vi "GetProbePlanCoordinates.vi"(8 "Use index as X coord":bool=TRUE, 9 "Probe Card Channels":i32=1) -> (0 "file path":string, 2 "OK?":bool, 3 "Array":T1(array[cluster]))   [LabVIEW 2018] (continued)
\nLabel=Strip\t763\tX=19403.20\ty=17360.64 \nLabel=Strip\t764\tX=19749.10\ty=17461.35 \nLabel=Strip\t765\tX=19396.46\ty=17516.68 \nLabel=Strip\t766\tX=19742.32\ty=17617.52 \nLabel=Strip\t767\tX=19389.66\ty=17672.72 \nLabel=Strip\t768\tX=19735.48\ty=17773.69 \nLabel=Strip\t769\tX=19382.79\ty=17828.75 \nLabel=Strip\t770\tX=19728.58\ty=17929.86 \nLabel=Strip\t771\tX=19375.87\ty=17984.79 \nLabel=Strip\t772\tX=19721.61\ty=18086.03 \nLabel=Strip\t773\tX=19368.89\ty=18140.82 \nLabel=Strip\t774\tX=19714.59\ty=18242.20 \nLabel=Strip\t775\tX=19361.84\ty=18296.85 \nLabel=Strip\t776\tX=19707.51\ty=18398.36 \nLabel=Strip\t777\tX=19354.74\ty=18452.88 \nLabel=Strip\t778\tX=19700.36\ty=18554.52 \nLabel=Strip\t779\tX=19347.57\ty=18608.91 \nLabel=Strip\t780\tX=19693.16\ty=18710.69 \nLabel=Strip\t781\tX=19340.34\ty=18764.93 \nLabel=Strip\t782\tX=19685.89\ty=18866.85 \nLabel=Strip\t783\tX=19333.06\ty=18920.96 \nLabel=Strip\t784\tX=19678.57\ty=19023.00 \nLabel=Strip\t785\tX=19325.71\ty=19076.98 \nLabel=Strip\t786\tX=19671.18\ty=19179.16 \nLabel=Strip\t787\tX=19318.30\ty=19233.00 \nLabel=Strip\t788\tX=19663.73\ty=19335.32 \nLabel=Strip\t789\tX=19310.84\ty=19389.02 \nLabel=Strip\t790\tX=19656.23\ty=19491.47 \nLabel=Strip\t791\tX=19303.31\ty=19545.04 \nLabel=Strip\t792\tX=19648.66\ty=19647.62 \nLabel=Strip\t793\tX=19295.72\ty=19701.06 \nLabel=Strip\t794\tX=19641.03\ty=19803.77 \nLabel=Strip\t795\tX=19288.07\ty=19857.07 \nLabel=Strip\t796\tX=19633.34\ty=19959.92 \nLabel=Strip\t797\tX=19280.36\ty=20013.08 \nLabel=Strip\t798\tX=19625.59\ty=20116.07 \nLabel=Strip\t799\tX=19272.59\ty=20169.10 \nLabel=Strip\t800\tX=19617.78\ty=20272.22 \nLabel=Strip\t801\tX=19264.76\ty=20325.11 \nLabel=Strip\t802\tX=19609.91\ty=20428.36 \nLabel=Strip\t803\tX=19256.87\ty=20481.12 \nLabel=Strip\t804\tX=19601.98\ty=20584.50 \nLabel=Strip\t805\tX=19248.92\ty=20637.12 \nLabel=Strip\t806\tX=19593.99\ty=20740.64 \nLabel=Strip\t807\tX=19240.91\ty=20793.13 \nLabel=Strip\t808\tX=19585.94\ty=20896.78 \nLabel=Strip\t809\tX=19232.84\ty=20949.13 \nLabel=Strip\t810\tX=19577.83\ty=21052.92 \nLabel=Strip\t811\tX=19224.71\ty=21105.13 \nLabel=Strip\t812\tX=19569.66\ty=21209.05 \nLabel=Strip\t813\tX=19216.52\ty=21261.13 \nLabel=Strip\t814\tX=19561.43\ty=21365.19 \nLabel=Strip\t815\tX=19208.26\ty=21417.13 \nLabel=Strip\t816\tX=19553.13\ty=21521.32 \nLabel=Strip\t817\tX=19199.95\ty=21573.12 \nLabel=Strip\t818\tX=19544.78\ty=21677.45 \nLabel=Strip\t819\tX=19191.58\ty=21729.12 \nLabel=Strip\t820\tX=19536.37\ty=21833.58 \nLabel=Strip\t821\tX=19183.14\ty=21885.11 \nLabel=Strip\t822\tX=19527.89\ty=21989.70 \nLabel=Strip\t823\tX=19174.65\ty=22041.10 \nLabel=Strip\t824\tX=19519.36\ty=22145.83 \nLabel=Strip\t825\tX=19166.09\ty=22197.09 \nLabel=Strip\t826\tX=19510.76\ty=22301.95 \nLabel=Strip\t827\tX=19157.48\ty=22353.07 \nLabel=Strip\t828\tX=19502.11\ty=22458.07 \nLabel=Strip\t829\tX=19148.80\ty=22509.06 \nLabel=Strip\t830\tX=19493.39\ty=22614.18 \nLabel=Strip\t831\tX=19140.07\ty=22665.04 \nLabel=Strip\t832\tX=19484.61\ty=22770.30 \nLabel=Strip\t833\tX=19131.27\ty=22821.02 \nLabel=Strip\t834\tX=19475.77\ty=22926.41 \nLabel=Strip\t835\tX=19122.41\ty=22976.99 \nLabel=Strip\t836\tX=19466.88\ty=23082.52 \nLabel=Strip\t837\tX=19113.50\ty=23132.97 \nLabel=Strip\t838\tX=19457.92\ty=23238.63 \nLabel=Strip\t839\tX=19104.52\ty=23288.94 \nLabel=Strip\t840\tX=19448.90\ty=23394.74 \nLabel=Strip\t841\tX=19095.48\ty=23444.91 \nLabel=Strip\t842\tX=19439.82\ty=23550.84 \nLabel=Strip\t843\tX=19086.38\ty=23600.88 \nLabel=Strip\t844\tX=19430.68\ty=23706.95 \nLabel=Strip\t845\tX=19077.22\ty=23756.85 \nLabel=Strip\t846\tX=19421.48\ty=23863.05 \nLabel=Strip\t847\tX=19068.01\ty=23912.81 \nLabel=Strip\t848\tX=19412.22\ty=24019.14 \nLabel=Strip\t849\tX=19058.73\ty=24068.78 \nLabel=Strip\t850\tX=19402.90\ty=24175.24 \nLabel=Strip\t851\tX=19049.39\ty=24224.74 \nLabel=Strip\t852\tX=19393.52\ty=24331.33 \nLabel=Strip\t853\tX=19039.99\ty=24380.69 \nLabel=Strip\t854\tX=19384.08\ty=24487.42 \nLabel=Strip\t855\tX=19030.52\ty=24536.65 \nLabel=Strip\t856\tX=19374.58\ty=24643.51 \nLabel=Strip\t857\tX=19021.00\ty=24692.60 \nLabel=Strip\t858\tX=19365.01\ty=24799.60 \nLabel=Strip\t859\tX=19011.42\ty=24848.55 \nLabel=Strip\t860\tX=19355.39\ty=24955.68 \nLabel=Strip\t861\tX=19001.78\ty=25004.50 \nLabel=Strip\t862\tX=19345.71\ty=25111.76 \nLabel=Strip\t863\tX=18992.08\ty=25160.44 \nLabel=Strip\t864\tX=19335.96\ty=25267.84 \nLabel=Strip\t865\tX=18982.31\ty=25316.39 \nLabel=Strip\t866\tX=19326.16\ty=25423.92 \nLabel=Strip\t867\tX=18972.49\ty=25472.33 \nLabel=Strip\t868\tX=19316.30\ty=25579.99 \nLabel=Strip\t869\tX=18962.61\ty=25628.27 \nLabel=Strip\t870\tX=19306.37\ty=25736.06 \nLabel=Strip\t871\tX=18952.66\ty=25784.20 \nLabel=Strip\t872\tX=19296.38\ty=25892.13 \nLabel=Strip\t873\tX=18942.66\ty=25940.13 \nLabel=Strip\t874\tX=19286.34\ty=26048.20 \nLabel=Strip\t875\tX=18932.59\ty=26096.06 \nLabel=Strip\t876\tX=19276.23\ty=26204.26 \nLabel=Strip\t877\tX=18922.47\ty=26251.99 \nLabel=Strip\t878\tX=19266.06\ty=26360.32 \nLabel=Strip\t879\tX=18912.28\ty=26407.92 \nLabel=Strip\t880\tX=19255.84\ty=26516.38 \nLabel=Strip\t881\tX=18902.04\ty=26563.84 \nLabel=Strip\t882\tX=19245.55\ty=26672.44 \nLabel=Strip\t883\tX=18891.73\ty=26719.76 \nLabel=Strip\t884\tX=19235.20\ty=26828.49 \nLabel=Strip\t885\tX=18881.36\ty=26875.68 \nLabel=Strip\t886\tX=19224.79\ty=26984.54 \nLabel=Strip\t887\tX=18870.94\ty=27031.59 \nLabel=Strip\t888\tX=19214.32\ty=27140.59 \nLabel=Strip\t889\tX=18860.45\ty=27187.50 \nLabel=Strip\t890\tX=19203.79\ty=27296.63 \nLabel=Strip\t891\tX=18849.90\ty=27343.41 \nLabel=Strip\t892\tX=19193.20\ty=27452.68 \nLabel=Strip\t893\tX=18839.29\ty=27499.32 \nLabel=Strip\t894\tX=19182.55\ty=27608.72 \nLabel=Strip\t895\tX=18828.62\ty=27655.22 \nLabel=Strip\t896\tX=19171.84\ty=27764.75 \nLabel=Strip\t897\tX=18817.90\ty=27811.12 \nLabel=Strip\t898\tX=19161.07\ty=27920.79 \nLabel=Strip\t899\tX=18807.11\ty=27967.02 \nLabel=Strip\t900\tX=19150.24\ty=28076.82 \nLabel=Strip\t901\tX=18796.26\ty=28122.91 \nLabel=Strip\t902\tX=19139.34\ty=28232.84 \nLabel=Strip\t903\tX=18785.35\ty=28278.80 \nLabel=Strip\t904\tX=19128.39\ty=28388.87 \nLabel=Strip\t905\tX=18774.37\ty=28434.69 \nLabel=Strip\t906\tX=19117.38\ty=28544.89 \nLabel=Strip\t907\tX=18763.34\ty=28590.58 \nLabel=Strip\t908\tX=19106.30\ty=28700.91 \nLabel=Strip\t909\tX=18752.25\ty=28746.46 \nLabel=Strip\t910\tX=19095.17\ty=28856.93 \nLabel=Strip\t911\tX=18741.10\ty=28902.34 \nLabel=Strip\t912\tX=19083.97\ty=29012.94 \nLabel=Strip\t913\tX=18729.89\ty=29058.22 \nLabel=Strip\t914\tX=19072.72\ty=29168.95 \nLabel=Strip\t915\tX=18718.61\ty=29214.09 \nLabel=Strip\t916\tX=19061.40\ty=29324.95 \nLabel=Strip\t917\tX=18707.28\ty=29369.96 \nLabel=Strip\t918\tX=19050.03\ty=29480.96 \nLabel=Strip\t919\tX=18695.89\ty=29525.83 \nLabel=Strip\t920\tX=19038.59\ty=29636.96 \nLabel=Strip\t921\tX=18684.43\ty=29681.70 \nLabel=Strip\t922\tX=19027.09\ty=29792.96 \nLabel=Strip\t923\tX=18672.92\ty=29837.56 \nLabel=Strip\t924\tX=19015.53\ty=29948.95 \nLabel=Strip\t925\tX=18661.34\ty=29993.41 \nLabel=Strip\t926\tX=19003.92\ty=30104.94 \nLabel=Strip\t927\tX=18649.71\ty=30149.27 \nLabel=Strip\t928\tX=18992.24\ty=30260.93 \nLabel=Strip\t929\tX=18638.01\ty=30305.12 \nLabel=Strip\t930\tX=18980.50\ty=30416.91 \nLabel=Strip\t931\tX=18626.26\ty=30460.97 \nLabel=Strip\t932\tX=18968.70\ty=30572.90 \nLabel=Strip\t933\tX=18614.44\ty=30616.81 \nLabel=Strip\t934\tX=18956.84\ty=30728.87 \nLabel=Strip\t935\tX=18602.56\ty=30772.66 \nLabel=Strip\t936\tX=18944.92\ty=30884.85 \nLabel=Strip\t937\tX=18590.63\ty=30928.50 \nLabel=Strip\t938\tX=18932.94\ty=31040.82 \nLabel=Strip\t939\tX=18578.63\ty=31084.33 \nLabel=Strip\t940\tX=18920.90\ty=31196.79 \nLabel=Strip\t941\tX=18566.57\ty=31240.16 \nLabel=Strip\t942\tX=18908.80\ty=31352.75 \nLabel=Strip\t943\tX=18554.45\ty=31395.99 \nLabel=Strip\t944\tX=18896.63\ty=31508.71 \nLabel=Strip\t945\tX=18542.27\ty=31551.82 \nLabel=Strip\t946\tX=18884.41\ty=31664.67 \nLabel=Strip\t947\tX=18530.03\ty=31707.64 \nLabel=Strip\t948\tX=18872.13\ty=31820.63 \nLabel=Strip\t949\tX=18517.73\ty=31863.46 \nLabel=Strip\t950\tX=18859.79\ty=31976.58 \nLabel=Strip\t951\tX=18505.37\ty=32019.27 \nLabel=Strip\t952\tX=18847.38\ty=32132.53 \nLabel=Strip\t953\tX=18492.95\ty=32175.08 \nLabel=Strip\t954\tX=18834.92\ty=32288.47 \nLabel=Strip\t955\tX=18480.47\ty=32330.89 \nLabel=Strip\t956\tX=18822.39\ty=32444.41 \nLabel=Strip\t957\tX=18467.93\ty=32486.69 \nLabel=Strip\t958\tX=18809.81\ty=32600.35 \nLabel=Strip\t959\tX=18455.33\ty=32642.50 \nLabel=Strip\t960\tX=18797.16\ty=32756.28 \nLabel=Strip\t961\tX=18442.67\ty=32798.29 \nLabel=Strip\t962\tX=18784.46\ty=32912.21 \nLabel=Strip\t963\tX=18429.95\ty=32954.09 \nLabel=Strip\t964\tX=18771.69\ty=33068.14 \nLabel=Strip\t965\tX=18417.16\ty=33109.88 \nLabel=Strip\t966\tX=18758.86\ty=33224.06 \nLabel=Strip\t967\tX=18404.32\ty=33265.66 \nLabel=Strip\t968\tX=18745.97\ty=33379.98 \nLabel=Strip\t969\tX=18391.42\ty=33421.45 \nLabel=Strip\t970\tX=18733.03\ty=33535.89 \nLabel=Strip\t971\tX=18378.45\ty=33577.22 \nLabel=Strip\t972\tX=18720.02\ty=33691.81 \nLabel=Strip\t973\tX=18365.43\ty=33733.00 \nLabel=Strip\t974\tX=18706.95\ty=33847.71 \nLabel=Strip\t975\tX=18352.34\ty=33888.77 \nLabel=Strip\t976\tX=18693.82\ty=34003.62 \nLabel=Strip\t977\tX=18339.20\ty=34044.54 \nLabel=Strip\t978\tX=18680.63\ty=34159.52 \nLabel=Strip\t979\tX=18325.99\ty=34200.30 \nLabel=Strip\t980\tX=18667.38\ty=34315.41 \nLabel=Strip\t981\tX=18312.73\ty=34356.06 \nLabel=Strip\t982\tX=18654.07\ty=34471.31 \nLabel=Strip\t983\tX=18299.40\ty=34511.82 \nLabel=Strip\t984\tX=18640.70\ty=34627.19 \nLabel=Strip\t985\tX=18286.01\ty=34667.57 \nLabel=Strip\t986\tX=18627.27\ty=34783.08 \nLabel=Strip\t987\tX=18272.57\ty=34823.32 \nLabel=Strip\t988\tX=18613.78\ty=34938.96 \nLabel=Strip\t989\tX=18259.06\ty=34979.06 \nLabel=Strip\t990\tX=18600.22\ty=35094.84 \nLabel=Strip\t991\tX=18245.49\ty=35134.80 \nLabel=Strip\t992\tX=18586.61\ty=35250.71 \nLabel=Strip\t993\tX=18231.86\ty=35290.54 \nLabel=Strip\t994\tX=18572.94\ty=35406.58 \nLabel=Strip\t995\tX=18218.17\ty=35446.27 \nLabel=Strip\t996\tX=18559.20\ty=35562.44 \nLabel=Strip\t997\tX=18204.42\ty=35602.00 \nLabel=Strip\t998\tX=18545.41\ty=35718.30 \nLabel=Strip\t999\tX=18190.61\ty=35757.73 \nLabel=Strip\t1000\tX=18531.55\ty=35874.16 \nLabel=Strip\t1001\tX=18176.74\ty=35913.45 \nLabel=Strip\t1002\tX=18517.64\ty=36030.01 \nLabel=Strip\t1003\tX=18162.81\ty=36069.16 \nLabel=Strip\t1004\tX=18503.66\ty=36185.86 \nLabel=Strip\t1005\tX=18148.82\ty=36224.87 \nLabel=Strip\t1006\tX=18489.63\ty=36341.71 \nLabel=Strip\t1007\tX=18134.77\ty=36380.58 \nLabel=Strip\t1008\tX=18475.53\ty=36497.55 \nLabel=Strip\t1009\tX=18120.66\ty=36536.29 \nLabel=Strip\t1010\tX=18461.38\ty=36653.38 \nLabel=Strip\t1011\tX=18106.49\ty=36691.99 \nLabel=Strip\t1012\tX=18447.16\ty=36809.21 \nLabel=Strip\t1013\tX=18092.26\ty=36847.68 \nLabel=Strip\t1014\tX=18432.88\ty=36965.04 \nLabel=Strip\t1015\tX=18077.96\ty=37003.37 \nLabel=Strip\t1016\tX=18418.54\ty=37120.87 \nLabel=Strip\t1017\tX=18063.61\ty=37159.06 \nLabel=Strip\t1018\tX=18404.14\ty=37276.69 \nLabel=Strip\t1019\tX=18049.20\ty=37314.74 \nLabel=Strip\t1020\tX=18389.68\ty=37432.50 \nLabel=Strip\t1021\tX=18034.72\ty=37470.42 \nLabel=Strip\t1022\tX=18375.17\ty=37588.31 \nLabel=Strip\t1023\tX=18020.19\ty=37626.10 \nLabel=Strip\t1024\tX=18360.59\ty=37744.12 \nLabel=Strip\t1025\tX=18005.60\ty=37781.77 \nLabel=Strip\t1026\tX=18345.95\ty=37899.92 \nRegion=Segment\t2T\nLabel=Strip\t1\tX=39999.81\ty=-43820.71 \nLabel=Strip\t2\tX=40357.07\ty=-43767.72 \nLabel=Strip\t3\tX=40016.67\ty=-43657.21 \nLabel=Strip\t4\tX=40373.91\ty=-43604.08 \nLabel=Strip\t5\tX=40033.47\ty=-43493.70 \nLabel=Strip\t6\tX=40390.68\ty=-43440.44 \nLabel=Strip\t7\tX=40050.20\ty=-43330.19 \nLabel=Strip\t8\tX=40407.40\ty=-43276.78 \nLabel=Strip\t9\tX=40066.88\ty=-43166.67 \nLabel=Strip\t10\tX=40424.05\ty=-43113.12 \nLabel=Strip\t11\tX=40083.48\ty=-43003.14 \nLabel=Strip\t12\tX=40440.64\ty=-42949.45 \nLabel=Strip\t13\tX=40100.03\ty=-42839.60 \nLabel=Strip\t14\tX=40457.16\ty=-42785.78 \nLabel=Strip\t15\tX=40116.51\ty=-42676.05 \nLabel=Strip\t16\tX=40473.62\ty=-42622.09 \nLabel=Strip\t17\tX=40132.93\ty=-42512.50 \nLabel=Strip\t18\tX=40490.02\ty=-42458.40 \nLabel=Strip\t19\tX=40149.29\ty=-42348.94 \nLabel=Strip\t20\tX=40506.35\ty=-42294.70 \nLabel=Strip\t21\tX=40165.58\ty=-42185.37 \nLabel=Strip\t22\tX=40522.63\ty=-42130.99 \nLabel=Strip\t23\tX=40181.81\ty=-42021.79 \nLabel=Strip\t24\tX=40538.84\ty=-41967.28 \nLabel=Strip\t25\tX=40197.98\ty=-41858.21 \nLabel=Strip\t26\tX=40554.98\ty=-41803.56 \nLabel=Strip\t27\tX=40214.08\ty=-41694.62 \nLabel=Strip\t28\tX=40571.07\ty=-41639.83 \nLabel=Strip\t29\tX=40230.13\ty=-41531.02 \nLabel=Strip\t30\tX=40587.09\ty=-41476.09 \nLabel=Strip\t31\tX=40246.10\ty=-41367.41 \nLabel=Strip\t32\tX=40603.05\ty=-41312.34 \nLabel=Strip\t33\tX=40262.02\ty=-41203.80 \nLabel=Strip\t34\tX=40618.94\ty=-41148.59 \nLabel=Strip\t35\tX=40277.87\ty=-41040.18 \nLabel=Strip\t36\tX=40634.77\ty=-40984.83 \nLabel=Strip\t37\tX=40293.66\ty=-40876.55 \nLabel=Strip\t38\tX=40650.54\ty=-40821.07 \nLabel=Strip\t39\tX=40309.39\ty=-40712.91 \nLabel=Strip\t40\tX=40666.25\ty=-40657.29 \nLabel=Strip\t41\tX=40325.05\ty=-40549.27 \nLabel=Strip\t42\tX=40681.89\ty=-40493.51 \nLabel=Strip\t43\tX=40340.65\ty=-40385.62 \nLabel=Strip\t44\tX=40697.47\ty=-40329.72 \nLabel=Strip\t45\tX=40356.19\ty=-40221.96 \nLabel=Strip\t46\tX=40712.99\ty=-40165.92 \nLabel=Strip\t47\tX=40371.67\ty=-40058.29 \nLabel=Strip\t48\tX=40728.44\ty=-40002.12 \nLabel=Strip\t49\tX=40387.08\ty=-39894.62 \nLabel=Strip\t50\tX=40743.83\ty=-39838.31 \nLabel=Strip\t51\tX=40402.43\ty=-39730.94 \nLabel=Strip\t52\tX=40759.16\ty=-39674.49 \nLabel=Strip\t53\tX=40417.72\ty=-39567.26 \nLabel=Strip\t54\tX=40774.42\ty=-39510.67 \nLabel=Strip\t55\tX=40432.94\ty=-39403.56 \nLabel=Strip\t56\tX=40789.62\ty=-39346.83 \nLabel=Strip\t57\tX=40448.10\ty=-39239.86 \nLabel=Strip\t58\tX=40804.76\ty=-39182.99 \nLabel=Strip\t59\tX=40463.20\ty=-39076.15 \nLabel=Strip\t60\tX=40819.84\ty=-39019.15 \nLabel=Strip\t61\tX=40478.23\ty=-38912.44 \nLabel=Strip\t62\tX=40834.85\ty=-38855.29 \nLabel=Strip\t63\tX=40493.20\ty=-38748.71 \nLabel=Strip\t64\tX=40849.80\ty=-38691.43 \nLabel=Strip\t65\tX=40508.11\ty=-38584.98 \nLabel=Strip\t66\tX=40864.69\ty=-38527.56 \nLabel=Strip\t67\tX=40522.96\ty=-38421.25 \nLabel=Strip\t68\tX=40879.51\ty=-38363.69 \nLabel=Strip\t69\tX=40537.74\ty=-38257.50 \nLabel=Strip\t70\tX=40894.27\ty=-38199.81 \nLabel=Strip\t71\tX=40552.46\ty=-38093.75 \nLabel=Strip\t72\tX=40908.97\ty=-38035.92 \nLabel=Strip\t73\tX=40567.11\ty=-37930.00 \nLabel=Strip\t74\tX=40923.60\ty=-37872.02 \nLabel=Strip\t75\tX=40581.71\ty=-37766.23 \nLabel=Strip\t76\tX=40938.17\ty=-37708.12 \nLabel=Strip\t77\tX=40596.24\ty=-37602.46 \nLabel=Strip\t78\tX=40952.68\ty=-37544.21 \nLabel=Strip\t79\tX=40610.70\ty=-37438.68 \nLabel=Strip\t80\tX=40967.12\ty=-37380.29 \nLabel=Strip\t81\tX=40625.11\ty=-37274.90 \nLabel=Strip\t82\tX=40981.50\ty=-37216.37 \nLabel=Strip\t83\tX=40639.45\ty=-37111.10 \nLabel=Strip\t84\tX=40995.82\ty=-37052.44 \nLabel=Strip\t85\tX=40653.73\ty=-36947.31 \nLabel=Strip\t86\tX=41010.08\ty=-36888.50 \nLabel=Strip\t87\tX=40667.94\ty=-36783.50 \nLabel=Strip\t88\tX=41024.27\ty=-36724.56 \nLabel=Strip\t89\tX=40682.09\ty=-36619.69 \nLabel=Strip\t90\tX=41038.40\ty=-36560.61 \nLabel=Strip\t91\tX=40696.18\ty=-36455.87 \nLabel=Strip\t92\tX=41052.47\ty=-36396.65 \nLabel=Strip\t93\tX=40710.21\ty=-36292.04 \nLabel=Strip\t94\tX=41066.47\ty=-36232.69 \nLabel=Strip\t95\tX=40724.17\ty=-36128.21 \nLabel=Strip\t96\tX=41080.41\ty=-36068.72 \nLabel=Strip\t97\tX=40738.07\ty=-35964.37 \nLabel=Strip\t98\tX=41094.29\ty=-35904.74 \nLabel=Strip\t99\tX=40751.91\ty=-35800.52 \nLabel=Strip\t100\tX=41108.10\ty=-35740.75 \nLabel=Strip\t101\tX=40765.68\ty=-35636.67 \nLabel=Strip\t102\tX=41121.85\ty=-35576.76 \nLabel=Strip\t103\tX=40779.39\ty=-35472.81 \nLabel=Strip\t104\tX=41135.54\ty=-35412.77 \nLabel=Strip\t105\tX=40793.04\ty=-35308.95 \nLabel=Strip\t106\tX=41149.16\ty=-35248.76 \nLabel=Strip\t107\tX=40806.62\ty=-35145.07 \nLabel=Strip\t108\tX=41162.72\ty=-35084.75 \nLabel=Strip\t109\tX=40820.14\ty=-34981.20 \nLabel=Strip\t110\tX=41176.22\ty=-34920.73 \nLabel=Strip\t111\tX=40833.60\ty=-34817.31 \nLabel=Strip\t112\tX=41189.66\ty=-34756.71 \nLabel=Strip\t113\tX=40847.00\ty=-34653.42 \nLabel=Strip\t114\tX=41203.03\ty=-34592.68 \nLabel=Strip\t115\tX=40860.33\ty=-34489.52 \nLabel=Strip\t116\tX=41216.34\ty=-34428.64 \nLabel=Strip\t117\tX=40873.60\ty=-34325.62 \nLabel=Strip\t118\tX=41229.58\ty=-34264.60 \nLabel=Strip\t119\tX=40886.80\ty=-34161.71 \nLabel=Strip\t120\tX=41242.76\ty=-34100.55 \nLabel=Strip\t121\tX=40899.95\ty=-33997.79 \nLabel=Strip\t122\tX=41255.88\ty=-33936.50 \nLabel=Strip\t123\tX=40913.03\ty=-33833.86 \nLabel=Strip\t124\tX=41268.94\ty=-33772.44 \nLabel=Strip\t125\tX=40926.04\ty=-33669.93 \nLabel=Strip\t126\tX=41281.93\ty=-33608.37 \nLabel=Strip\t127\tX=40938.99\ty=-33506.12 \nLabel=Strip\t128\tX=41294.86\ty=-33444.29 \nLabel=Strip\t129\tX=40951.89\ty=-33342.05 \nLabel=Strip\t130\tX=41307.73\ty=-33280.21 \nLabel=Strip\t131\tX=40964.71\ty=-33178.11 \nLabel=Strip\t132\tX=41320.53\ty=-33116.12 \nLabel=Strip\t133\tX=40977.48\ty=-33014.15 \nLabel=Strip\t134\tX=41333.27\ty=-32952.03 \nLabel=Strip\t135\tX=40990.18\ty=-32850.19 \nLabel=Strip\t136\tX=41345.95\ty=-32787.93 \nLabel=Strip\t137\tX=41002.81\ty=-32686.22 \nLabel=Strip\t138\tX=41358.56\ty=-32623.83 \nLabel=Strip\t139\tX=41015.39\ty=-32522.25 \nLabel=Strip\t140\tX=41371.11\ty=-32459.71 \nLabel=Strip\t141\tX=41027.90\ty=-32358.27 \nLabel=Strip\t142\tX=41383.60\ty=-32295.60 \nLabel=Strip\t143\tX=41040.35\ty=-32194.28 \nLabel=Strip\t144\tX=41396.02\ty=-32131.47 \nLabel=Strip\t145\tX=41052.73\ty=-32030.29 \nLabel=Strip\t146\tX=41408.38\ty=-31967.34 \nLabel=Strip\t147\tX=41065.05\ty=-31866.29 \nLabel=Strip\t148\tX=41420.68\ty=-31803.21 \nLabel=Strip\t149\tX=41077.31\ty=-31702.29 \nLabel=Strip\t150\tX=41432.91\ty=-31639.06 \nLabel=Strip\t151\tX=41089.51\ty=-31538.28 \nLabel=Strip\t152\tX=41445.09\ty=-31474.92 \nLabel=Strip\t153\tX=41101.64\ty=-31374.26 \nLabel=Strip\t154\tX=41457.19\ty=-31310.76 \nLabel=Strip\t155\tX=41113.71\ty=-31210.24 \nLabel=Strip\t156\tX=41469.24\ty=-31146.60 \nLabel=Strip\t157\tX=41125.72\ty=-31046.21 \nLabel=Strip\t158\tX=41481.22\ty=-30982.44 \nLabel=Strip\t159\tX=41137.66\ty=-30882.18 \nLabel=Strip\t160\tX=41493.14\ty=-30818.26 \nLabel=Strip\t161\tX=41149.54\ty=-30718.14 \nLabel=Strip\t162\tX=41504.99\ty=-30654.09 \nLabel=Strip\t163\tX=41161.36\ty=-30554.09 \nLabel=Strip\t164\tX=41516.79\ty=-30489.90 \nLabel=Strip\t165\tX=41173.11\ty=-30390.04 \nLabel=Strip\t166\tX=41528.51\ty=-30325.71 \nLabel=Strip\t167\tX=41184.80\ty=-30225.98 \nLabel=Strip\t168\tX=41540.18\ty=-30161.52 \nLabel=Strip\t169\tX=41196.43\ty=-30061.92 \nLabel=Strip\t170\tX=41551.78\ty=-29997.32 \nLabel=Strip\t171\tX=41207.99\ty=-29897.85 \nLabel=Strip\t172\tX=41563.32\ty=-29833.11 \nLabel=Strip\t173\tX=41219.49\ty=-29733.77 \nLabel=Strip\t174\tX=41574.80\ty=-29668.90 \nLabel=Strip\t175\tX=41230.93\ty=-29569.69 \nLabel=Strip\t176\tX=41586.21\ty=-29504.68 \nLabel=Strip\t177\tX=41242.30\ty=-29405.61 \nLabel=Strip\t178\tX=41597.56\ty=-29340.45 \nLabel=Strip\t179\tX=41253.61\ty=-29241.51 \nLabel=Strip\t180\tX=41608.84\ty=-29176.22 \nLabel=Strip\t181\tX=41264.86\ty=-29077.42 \nLabel=Strip\t182\tX=41620.07\ty=-29011.99 \nLabel=Strip\t183\tX=41276.05\ty=-28913.31 \nLabel=Strip\t184\tX=41631.23\ty=-28847.75 \nLabel=Strip\t185\tX=41287.17\ty=-28749.21 \nLabel=Strip\t186\tX=41642.32\ty=-28683.50 \nLabel=Strip\t187\tX=41298.23\ty=-28585.09 \nLabel=Strip\t188\tX=41653.36\ty=-28519.25 \nLabel=Strip\t189\tX=41309.22\ty=-28420.97 \nLabel=Strip\t190\tX=41664.33\ty=-28354.99 \nLabel=Strip\t191\tX=41320.15\ty=-28256.84 \nLabel=Strip\t192\tX=41675.23\ty=-28190.73 \nLabel=Strip\t193\tX=41331.02\ty=-28092.71 \nLabel=Strip\t194\tX=41686.07\ty=-28026.46 \nLabel=Strip\t195\tX=41341.83\ty=-27928.58 \nLabel=Strip\t196\tX=41696.85\ty=-27862.18 \nLabel=Strip\t197\tX=41352.57\ty=-27764.44 \nLabel=Strip\t198\tX=41707.57\ty=-27697.90 \nLabel=Strip\t199\tX=41363.25\ty=-27600.29 \nLabel=Strip\t200\tX=41718.22\ty=-27533.62 \nLabel=Strip\t201\tX=41373.86\ty=-27436.13 \nLabel=Strip\t202\tX=41728.81\ty=-27369.33 \nLabel=Strip\t203\tX=41384.42\ty=-27271.98 \nLabel=Strip\t204\tX=41739.34\ty=-27205.03 \nLabel=Strip\t205\tX=41394.90\ty=-27107.81 \nLabel=Strip\t206\tX=41749.80\ty=-27040.73 \nLabel=Strip\t207\tX=41405.33\ty=-26943.64 \nLabel=Strip\t208\tX=41760.20\ty=-26876.42 \nLabel=Strip\t209\tX=41415.69\ty=-26779.47 \nLabel=Strip\t210\tX=41770.54\ty=-26712.11 \nLabel=Strip\t211\tX=41425.99\ty=-26615.29 \nLabel=Strip\t212\tX=41780.81\ty=-26547.80 \nLabel=Strip\t213\tX=41436.23\ty=-26451.11 \nLabel=Strip\t214\tX=41791.02\ty=-26383.47 \nLabel=Strip\t215\tX=41446.40\ty=-26286.92 \nLabel=Strip\t216\tX=41801.17\ty=-26219.15 \nLabel=Strip\t217\tX=41456.51\ty=-26122.72 \nLabel=Strip\t218\tX=41811.25\ty=-26054.81 \nLabel=Strip\t219\tX=41466.56\ty=-25958.52 \nLabel=Strip\t220\tX=41821.27\ty=-25890.47 \nLabel=Strip\t221\tX=41476.54\ty=-25794.31 \nLabel=Strip\t222\tX=41831.23\ty=-25726.13 \nLabel=Strip\t223\tX=41486.46\ty=-25630.10 \nLabel=Strip\t224\tX=41841.12\ty=-25561.78 \nLabel=Strip\t225\tX=41496.32\ty=-25465.89 \nLabel=Strip\t226\tX=41850.95\ty=-25397.43 \nLabel=Strip\t227\tX=41506.11\ty=-25301.67 \nLabel=Strip\t228\tX=41860.72\ty=-25233.07 \nLabel=Strip\t229\tX=41515.84\ty=-25137.44 \nLabel=Strip\t230\tX=41870.42\ty=-25068.71 \nLabel=Strip\t231\tX=41525.51\ty=-24973.21 \nLabel=Strip\t232\tX=41880.06\ty=-24904.34 \nLabel=Strip\t233\tX=41535.11\ty=-24808.97 \nLabel=Strip\t234\tX=41889.64\ty=-24739.96 \nLabel=Strip\t235\tX=41544.65\ty=-24644.73 \nLabel=Strip\t236\tX=41899.16\ty=-24575.59 \nLabel=Strip\t237\tX=41554.13\ty=-24480.49 \nLabel=Strip\t238\tX=41908.61\ty=-24411.20 \nLabel=Strip\t239\tX=41563.54\ty=-24316.24 \nLabel=Strip\t240\tX=41917.99\ty=-24246.81 \nLabel=Strip\t241\tX=41572.89\ty=-24151.98 \nLabel=Strip\t242\tX=41927.32\ty=-24082.42 \nLabel=Strip\t243\tX=41582.18\ty=-23987.72 \nLabel=Strip\t244\tX=41936.57\ty=-23918.02 \nLabel=Strip\t245\tX=41591.40\ty=-23823.45 \nLabel=Strip\t246\tX=41945.77\ty=-23753.62 \nLabel=Strip\t247\tX=41600.56\ty=-23659.18 \nLabel=Strip\t248\tX=41954.92\ty=-23588.64 \nLabel=Strip\t249\tX=41609.66\ty=-23494.91 \nLabel=Strip\t250\tX=41963.98\ty=-23424.80 \nLabel=Strip\t251\tX=41618.69\ty=-23330.63 \nLabel=Strip\t252\tX=41972.98\ty=-23260.38 \nLabel=Strip\t253\tX=41627.66\ty=-23166.34 \nLabel=Strip\t254\tX=41981.92\ty=-23095.96 \nLabel=Strip\t255\tX=41636.57\ty=-23002.05 \nLabel=Strip\t256\tX=41990.81\ty=-22931.53 \nLabel=Strip\t257\tX=41645.41\ty=-22837.76 \nLabel=Strip\t258\tX=41999.62\ty=-22767.10 \nLabel=Strip\t259\tX=41654.19\ty=-22673.46 \nLabel=Strip\t260\tX=42008.37\ty=-22602.66 \nLabel=Strip\t261\tX=41662.91\ty=-22509.15 \nLabel=Strip\t262\tX=42017.06\ty=-22438.22 \nLabel=Strip\t263\tX=41671.56\ty=-22344.85 \nLabel=Strip\t264\tX=42025.69\ty=-22273.77 \nLabel=Strip\t265\tX=41680.15\ty=-22180.53 \nLabel=Strip\t266\tX=42034.25\ty=-22109.32 \nLabel=Strip\t267\tX=41688.68\ty=-22016.21 \nLabel=Strip\t268\tX=42042.75\ty=-21944.87 \nLabel=Strip\t269\tX=41697.14\ty=-21851.89 \nLabel=Strip\t270\tX=42051.19\ty=-21780.41 \nLabel=Strip\t271\tX=41705.54\ty=-21687.57 \nLabel=Strip\t272\tX=42059.56\ty=-21615.94 \nLabel=Strip\t273\tX=41713.88\ty=-21523.23 \nLabel=Strip\t274\tX=42067.87\ty=-21451.48 \nLabel=Strip\t275\tX=41722.16\ty=-21358.90 \nLabel=Strip\t276\tX=42076.12\ty=-21287.00 \nLabel=Strip\t277\tX=41730.37\ty=-21194.56 \nLabel=Strip\t278\tX=42084.30\ty=-21122.53 \nLabel=Strip\t279\tX=41738.51\ty=-21030.21 \nLabel=Strip\t280\tX=42092.42\ty=-20958.04 \nLabel=Strip\t281\tX=41746.60\ty=-20865.86 \nLabel=Strip\t282\tX=42100.48\ty=-20793.56 \nLabel=Strip\t283\tX=41754.62\ty=-20701.51 \nLabel=Strip\t284\tX=42108.47\ty=-20629.06 \nLabel=Strip\t285\tX=41762.57\ty=-20537.15 \nLabel=Strip\t286\tX=42116.40\ty=-20464.57 \nLabel=Strip\t287\tX=41770.47\ty=-20372.79 \nLabel=Strip\t288\tX=42124.26\ty=-20300.07 \nLabel=Strip\t289\tX=41778.30\ty=-20208.42 \nLabel=Strip\t290\tX=42132.06\ty=-20135.57 \nLabel=Strip\t291\tX=41786.06\ty=-20044.05 \nLabel=Strip\t292\tX=42139.80\ty=-19971.06 \nLabel=Strip\t293\tX=41793.77\ty=-19879.68 \nLabel=Strip\t294\tX=42147.48\ty=-19806.54 \nLabel=Strip\t295\tX=41801.41\ty=-19715.30 \nLabel=Strip\t296\tX=42155.09\ty=-19642.03 \nLabel=Strip\t297\tX=41808.98\ty=-19550.91 \nLabel=Strip\t298\tX=42162.64\ty=-19477.51 \nLabel=Strip\t299\tX=41816.50\ty=-19386.52 \nLabel=Strip\t300\tX=42170.12\ty=-19312.98 \nLabel=Strip\t301\tX=41823.95\ty=-19222.13 \nLabel=Strip\t302\tX=42177.54\ty=-19148.45 \nLabel=Strip\t303\tX=41831.33\ty=-19057.74 \nLabel=Strip\t304\tX=42184.90\ty=-18983.92 \nLabel=Strip\t305\tX=41838.66\ty=-18893.33 \nLabel=Strip\t306\tX=42192.20\ty=-18819.38 \nLabel=Strip\t307\tX=41845.92\ty=-18728.93 \nLabel=Strip\t308\tX=42199.43\ty=-18654.84 \nLabel=Strip\t309\tX=41853.11\ty=-18564.52 \nLabel=Strip\t310\tX=42206.60\ty=-18490.29 \nLabel=Strip\t311\tX=41860.25\ty=-18400.11 \nLabel=Strip\t312\tX=42213.70\ty=-18325.74 \nLabel=Strip\t313\tX=41867.32\ty=-18235.69 \nLabel=Strip\t314\tX=42220.74\ty=-18161.19 \nLabel=Strip\t315\tX=41874.32\ty=-18071.27 \nLabel=Strip\t316\tX=42227.72\ty=-17996.63 \nLabel=Strip\t317\tX=41881.26\ty=-17906.84 \nLabel=Strip\t318\tX=42234.63\ty=-17832.07 \nLabel=Strip\t319\tX=41888.14\ty=-17742.42 \nLabel=Strip\t320\tX=42241.48\ty=-17667.50 \nLabel=Strip\t321\tX=41894.96\ty=-17577.98 \nLabel=Strip\t322\tX=42248.27\ty=-17502.93 \nLabel=Strip\t323\tX=41901.71\ty=-17413.55 \nLabel=Strip\t324\tX=42254.99\ty=-17338.36 \nLabel=Strip\t325\tX=41908.40\ty=-17249.10 \nLabel=Strip\t326\tX=42261.65\ty=-17173.78 \nLabel=Strip\t327\tX=41915.03\ty=-17084.66 \nLabel=Strip\t328\tX=42268.25\ty=-17009.20 \nLabel=Strip\t329\tX=41921.59\ty=-16920.20 \nLabel=Strip\t330\tX=42274.78\ty=-16844.61 \nLabel=Strip\t331\tX=41928.09\ty=-16755.76 \nLabel=Strip\t332\tX=42281.25\ty=-16680.02 \nLabel=Strip\t333\tX=41934.52\ty=-16591.30 \nLabel=Strip\t334\tX=42287.66\ty=-16515.43 \nLabel=Strip\t335\tX=41940.90\ty=-16426.84 \nLabel=Strip\t336\tX=42294.00\ty=-16350.83 \nLabel=Strip\t337\tX=41947.21\ty=-16262.38 \nLabel=Strip\t338\tX=42300.28\ty=-16186.23 \nLabel=Strip\t339\tX=41953.45\ty=-16097.91 \nLabel=Strip\t340\tX=42306.50\ty=-16021.63 \nLabel=Strip\t341\tX=41959.63\ty=-15933.44 \nLabel=Strip\t342\tX=42312.65\ty=-15857.02 \nLabel=Strip\t343\tX=41965.75\ty=-15768.97 \nLabel=Strip\t344\tX=42318.74\ty=-15692.41 \nLabel=Strip\t345\tX=41971.80\ty=-15604.49 \nLabel=Strip\t346\tX=42324.76\ty=-15527.79 \nLabel=Strip\t347\tX=41977.80\ty=-15440.01 \nLabel=Strip\t348\tX=42330.73\ty=-15363.17 \nLabel=Strip\t349\tX=41983.72\ty=-15275.52 \nLabel=Strip\t350\tX=42336.62\ty=-15198.55 \nLabel=Strip\t351\tX=41989.59\ty=-15111.03 \nLabel=Strip\t352\tX=42342.46\ty=-15033.92 \nLabel=Strip\t353\tX=41995.39\ty=-14946.54 \nLabel=Strip\t354\tX=42348.23\ty=-14869.29 \nLabel=Strip\t355\tX=42001.13\ty=-14782.04 \nLabel=Strip\t356\tX=42353.94\ty=-14704.66 \nLabel=Strip\t357\tX=42006.80\ty=-14617.54 \nLabel=Strip\t358\tX=42359.58\ty=-14540.02 \nLabel=Strip\t359\tX=42012.41\ty=-14453.04 \nLabel=Strip\t360\tX=42365.16\ty=-14375.38 \nLabel=Strip\t361\tX=42017.96\ty=-14288.53 \nLabel=Strip\t362\tX=42370.68\ty=-14210.74 \nLabel=Strip\t363\tX=42023.44\ty=-14124.02 \nLabel=Strip\t364\tX=42376.13\ty=-14046.09 \nLabel=Strip\t365\tX=42028.86\ty=-13959.51 \nLabel=Strip\t366\tX=42381.53\ty=-13881.44 \nLabel=Strip\t367\tX=42034.22\ty=-13794.99 \nLabel=Strip\t368\tX=42386.85\ty=-13716.79 \nLabel=Strip\t369\tX=42039.51\ty=-13630.47 \nLabel=Strip\t370\tX=42392.12\ty=-13552.13 \nLabel=Strip\t371\tX=42044.74\ty=-13465.95 \nLabel=Strip\t372\tX=42397.32\ty=-13387.47 \nLabel=Strip\t373\tX=42049.91\ty=-13301.42 \nLabel=Strip\t374\tX=42402.45\ty=-13222.81 \nLabel=Strip\t375\tX=42055.01\ty=-13136.89 \nLabel=Strip\t376\tX=42407.52\ty=-13058.14 \nLabel=Strip\t377\tX=42060.05\ty=-12972.36 \nLabel=Strip\t378\tX=42412.53\ty=-12893.47 \nLabel=Strip\t379\tX=42065.03\ty=-12807.82 \nLabel=Strip\t380\tX=42417.48\ty=-12728.80 \nLabel=Strip\t381\tX=42069.94\ty=-12643.28 \nLabel=Strip\t382\tX=42422.36\ty=-12564.12 \nLabel=Strip\t383\tX=42074.79\ty=-12478.74 \nLabel=Strip\t384\tX=42427.18\ty=-12399.44 \nLabel=Strip\t385\tX=42079.58\ty=-12314.19 \nLabel=Strip\t386\tX=42431.94\ty=-12234.76 \nLabel=Strip\t387\tX=42084.30\ty=-12149.64 \nLabel=Strip\t388\tX=42436.63\ty=-12070.07 \nLabel=Strip\t389\tX=42088.96\ty=-11985.09 \nLabel=Strip\t390\tX=42441.26\ty=-11905.38 \nLabel=Strip\t391\tX=42093.55\ty=-11820.53 \nLabel=Strip\t392\tX=42445.82\ty=-11740.69 \nLabel=Strip\t393\tX=42098.09\ty=-11655.97 \nLabel=Strip\t394\tX=42450.32\ty=-11575.99 \nLabel=Strip\t395\tX=42102.55\ty=-11491.41 \nLabel=Strip\t396\tX=42454.76\ty=-11411.29 \nLabel=Strip\t397\tX=42106.96\ty=-11326.85 \nLabel=Strip\t398\tX=42459.13\ty=-11246.59 \nLabel=Strip\t399\tX=42111.30\ty=-11162.28 \nLabel=Strip\t400\tX=42463.44\ty=-11081.89 \nLabel=Strip\t401\tX=42115.58\ty=-10997.71 \nLabel=Strip\t402\tX=42467.69\ty=-10917.18 \nLabel=Strip\t403\tX=42119.79\ty=-10833.13 \nLabel=Strip\t404\tX=42471.87\ty=-10752.47 \nLabel=Strip\t405\tX=42124.03\ty=-10646.81 \nLabel=Strip\t406\tX=42476.06\ty=-10570.16 \nLabel=Strip\t407\tX=42128.08\ty=-10491.07 \nLabel=Strip\t408\tX=42480.08\ty=-10414.42 \nLabel=Strip\t409\tX=42132.07\ty=-10335.33 \nLabel=Strip\t410\tX=42484.04\ty=-10258.68 \nLabel=Strip\t411\tX=42136.00\ty=-10179.59 \nLabel=Strip\t412\tX=42487.94\ty=-10102.94 \nLabel=Strip\t413\tX=42139.87\ty=-10023.84 \nLabel=Strip\t414\tX=42491.78\ty=-9947.19 \nLabel=Strip\t415\tX=42143.68\ty=-9868.09 \nLabel=Strip\t416\tX=42495.63\ty=-9764.15 \nLabel=Strip\t417\tX=42147.51\ty=-9681.04 \nLabel=Strip\t418\tX=42499.37\ty=-9599.42 \nLabel=Strip\t419\tX=42151.22\ty=-9516.44 \nLabel=Strip\t420\tX=42503.05\ty=-9434.68 \nLabel=Strip\t421\tX=42154.86\ty=-9351.84 \nLabel=Strip\t422\tX=42506.66\ty=-9269.95 \nLabel=Strip\t423\tX=42158.44\ty=-9187.24 \nLabel=Strip\t424\tX=42510.21\ty=-9105.21 \nLabel=Strip\t425\tX=42161.96\ty=-9022.63 \nLabel=Strip\t426\tX=42513.69\ty=-8940.47 \nLabel=Strip\t427\tX=42165.41\ty=-8858.02 \nLabel=Strip\t428\tX=42517.11\ty=-8775.72 \nLabel=Strip\t429\tX=42168.80\ty=-8693.41 \nLabel=Strip\t430\tX=42520.47\ty=-8610.98 \nLabel=Strip\t431\tX=42172.12\ty=-8528.80 \nLabel=Strip\t432\tX=42523.76\ty=-8446.23 \nLabel=Strip\t433\tX=42175.38\ty=-8364.19 \nLabel=Strip\t434\tX=42526.99\ty=-8281.48 \nLabel=Strip\t435\tX=42178.58\ty=-8199.57 \nLabel=Strip\t436\tX=42530.16\ty=-8116.72 \nLabel=Strip\t437\tX=42181.72\ty=-8034.95 \nLabel=Strip\t438\tX=42533.26\ty=-7951.97 \nLabel=Strip\t439\tX=42184.79\ty=-7870.32 \nLabel=Strip\t440\tX=42536.30\ty=-7787.21 \nLabel=Strip\t441\tX=42187.79\ty=-7705.70 \nLabel=Strip\t442\tX=42539.27\ty=-7622.44 \nLabel=Strip\t443\tX=42190.74\ty=-7541.07 \nLabel=Strip\t444\tX=42542.18\ty=-7457.68 \nLabel=Strip\t445\tX=42193.62\ty=-7376.44 \nLabel=Strip\t446\tX=42545.03\ty=-7292.91 \nLabel=Strip\t447\tX=42196.43\ty=-7211.81 \nLabel=Strip\t448\tX=42547.82\ty=-7128.15 \nLabel=Strip\t449\tX=42199.19\ty=-7047.18 \nLabel=Strip\t450\tX=42550.54\ty=-6963.37 \nLabel=Strip\t451\tX=42201.88\ty=-6882.54 \nLabel=Strip\t452\tX=42553.19\ty=-6798.60 \nLabel=Strip\t453\tX=42204.50\ty=-6717.90 \nLabel=Strip\t454\tX=42555.79\ty=-6633.82 \nLabel=Strip\t455\tX=42207.07\ty=-6553.26 \nLabel=Strip\t456\tX=42558.32\ty=-6469.05 \nLabel=Strip\t457\tX=42209.56\ty=-6388.61 \nLabel=Strip\t458\tX=42560.78\ty=-6304.27 \nLabel=Strip\t459\tX=42212.00\ty=-6223.97 \nLabel=Strip\t460\tX=42563.19\ty=-6139.48 \nLabel=Strip\t461\tX=42214.37\ty=-6059.32 \nLabel=Strip\t462\tX=42565.53\ty=-5974.70 \nLabel=Strip\t463\tX=42216.68\ty=-5894.67 \nLabel=Strip\t464\tX=42567.80\ty=-5809.91 \nLabel=Strip\t465\tX=42218.92\ty=-5730.01 \nLabel=Strip\t466\tX=42570.01\ty=-5645.12 \nLabel=Strip\t467\tX=42221.11\ty=-5565.36 \nLabel=Strip\t468\tX=42572.16\ty=-5480.33 \nLabel=Strip\t469\tX=42223.22\ty=-5400.70 \nLabel=Strip\t470\tX=42574.25\ty=-5315.54 \nLabel=Strip\t471\tX=42225.28\ty=-5236.04 \nLabel=Strip\t472\tX=42576.27\ty=-5150.74 \nLabel=Strip\t473\tX=42227.27\ty=-5071.38 \nLabel=Strip\t474\tX=42578.22\ty=-4985.94 \nLabel=Strip\t475\tX=42229.19\ty=-4906.72 \nLabel=Strip\t476\tX=42580.12\ty=-4821.14 \nLabel=Strip\t477\tX=42231.06\ty=-4742.05 \nLabel=Strip\t478\tX=42581.95\ty=-4656.34 \nLabel=Strip\t479\tX=42232.86\ty=-4577.38 \nLabel=Strip\t480\tX=42583.71\ty=-4491.54 \nLabel=Strip\t481\tX=42234.59\ty=-4412.71 \nLabel=Strip\t482\tX=42585.42\ty=-4326.73 \nLabel=Strip\t483\tX=42236.27\ty=-4248.04 \nLabel=Strip\t484\tX=42587.06\ty=-4161.92 \nLabel=Strip\t485\tX=42237.87\ty=-4083.37 \nLabel=Strip\t486\tX=42588.63\ty=-3997.11 \nLabel=Strip\t487\tX=42239.42\ty=-3918.69 \nLabel=Strip\t488\tX=42590.14\ty=-3832.30 \nLabel=Strip\t489\tX=42240.90\ty=-3754.02 \nLabel=Strip\t490\tX=42591.59\ty=-3667.49 \nLabel=Strip\t491\tX=42242.32\ty=-3589.34 \nLabel=Strip\t492\tX=42592.98\ty=-3502.67 \nLabel=Strip\t493\tX=42243.67\ty=-3424.65 \nLabel=Strip\t494\tX=42594.30\ty=-3337.86 \nLabel=Strip\t495\tX=42244.96\ty=-3259.97 \nLabel=Strip\t496\tX=42595.56\ty=-3173.04 \nLabel=Strip\t497\tX=42246.19\ty=-3095.29 \nLabel=Strip\t498\tX=42596.75\ty=-3008.22 \nLabel=Strip\t499\tX=42247.36\ty=-2930.60 \nLabel=Strip\t500\tX=42597.88\ty=-2843.40 \nLabel=Strip\t501\tX=42248.46\ty=-2765.91 \nLabel=Strip\t502\tX=42598.95\ty=-2678.57 \nLabel=Strip\t503\tX=42249.49\ty=-2601.22 \nLabel=Strip\t504\tX=42599.95\ty=-2513.74 \nLabel=Strip\t505\tX=42250.47\ty=-2436.53 \nLabel=Strip\t506\tX=42600.89\ty=-2348.90 \nLabel=Strip\t507\tX=42251.37\ty=-2271.84 \nLabel=Strip\t508\tX=42601.76\ty=-2184.09 \nLabel=Strip\t509\tX=42252.22\ty=-2107.14 \nLabel=Strip\t510\tX=42602.58\ty=-2019.26 \nLabel=Strip\t511\tX=42253.00\ty=-1942.45 \nLabel=Strip\t512\tX=42603.32\ty=-1854.42 \nLabel=Strip\t513\tX=42253.72\ty=-1777.75 \nLabel=Strip\t514\tX=42604.01\ty=-1689.59 \nLabel=Strip\t515\tX=42254.38\ty=-1613.05 \nLabel=Strip\t516\tX=42604.63\ty=-1524.75 \nLabel=Strip\t517\tX=42254.97\ty=-1448.35 \nLabel=Strip\t518\tX=42605.19\ty=-1359.92 \nLabel=Strip\t519\tX=42255.49\ty=-1283.64 \nLabel=Strip\t520\tX=42605.68\ty=-1195.08 \nLabel=Strip\t521\tX=42255.96\ty=-1118.94 \nLabel=Strip\t522\tX=42606.11\ty=-1030.24 \nLabel=Strip\t523\tX=42256.36\ty=-954.23 \nLabel=Strip\t524\tX=42606.48\ty=-865.40 \nLabel=Strip\t525\tX=42256.70\ty=-789.53 \nLabel=Strip\t526\tX=42606.78\ty=-700.55 \nLabel=Strip\t527\tX=42256.97\ty=-624.82 \nLabel=Strip\t528\tX=42607.02\ty=-535.71 \nLabel=Strip\t529\tX=42257.18\ty=-460.11 \nLabel=Strip\t530\tX=42607.19\ty=-370.86 \nLabel=Strip\t531\tX=42257.32\ty=-295.40 \nLabel=Strip\t532\tX=42607.30\ty=-206.02 \nLabel=Strip\t533\tX=42257.41\ty=-130.68 \nLabel=Strip\t534\tX=42607.35\ty=-41.17 \nLabel=Strip\t535\tX=42257.43\ty=34.03 \nLabel=Strip\t536\tX=42607.34\ty=123.68 \nLabel=Strip\t537\tX=42257.38\ty=198.75 \nLabel=Strip\t538\tX=42607.26\ty=288.53 \nLabel=Strip\t539\tX=42257.27\ty=363.46 \nLabel=Strip\t540\tX=42607.11\ty=453.39 \nLabel=Strip\t541\tX=42257.10\ty=528.18 \nLabel=Strip\t542\tX=42606.91\ty=618.24 \nLabel=Strip\t543\tX=42256.87\ty=692.90 \nLabel=Strip\t544\tX=42606.64\ty=783.10 \nLabel=Strip\t545\tX=42256.57\ty=857.62 \nLabel=Strip\t546\tX=42606.30\ty=947.95 \nLabel=Strip\t547\tX=42256.20\ty=1022.34 \nLabel=Strip\t548\tX=42605.90\ty=1112.81 \nLabel=Strip\t549\tX=42255.78\ty=1187.06 \nLabel=Strip\t550\tX=42605.44\ty=1277.67 \nLabel=Strip\t551\tX=42255.29\ty=1351.79 \nLabel=Strip\t552\tX=42604.92\ty=1442.53 \nLabel=Strip\t553\tX=42254.73\ty=1516.51 \nLabel=Strip\t554\tX=42604.33\ty=1607.39 \nLabel=Strip\t555\tX=42254.11\ty=1681.24 \nLabel=Strip\t556\tX=42603.67\ty=1772.25 \nLabel=Strip\t557\tX=42253.43\ty=1845.97 \nLabel=Strip\t558\tX=42602.96\ty=1937.11 \nLabel=Strip\t559\tX=42252.69\ty=2010.69 \nLabel=Strip\t560\tX=42602.18\ty=2101.98 \nLabel=Strip\t561\tX=42251.88\ty=2175.42 \nLabel=Strip\t562\tX=42601.33\ty=2266.84 \nLabel=Strip\t563\tX=42251.01\ty=2340.15 \nLabel=Strip\t564\tX=42600.43\ty=2431.71 \nLabel=Strip\t565\tX=42250.07\ty=2504.89 \nLabel=Strip\t566\tX=42599.46\ty=2596.57 \nLabel=Strip\t567\tX=42249.07\ty=2669.62 \nLabel=Strip\t568\tX=42598.42\ty=2761.44 \nLabel=Strip\t569\tX=42248.01\ty=2834.35 \nLabel=Strip\t570\tX=42597.32\ty=2926.31 \nLabel=Strip\t571\tX=42246.88\ty=2999.08 \nLabel=Strip\t572\tX=42596.16\ty=3091.18 \nLabel=Strip\t573\tX=42245.69\ty=3163.82 \nLabel=Strip\t574\tX=42594.93\ty=3256.05 \nLabel=Strip\t575\tX=42244.44\ty=3328.56 \nLabel=Strip\t576\tX=42593.65\ty=3420.92 \nLabel=Strip\t577\tX=42243.12\ty=3493.29 \nLabel=Strip\t578\tX=42592.29\ty=3585.79 \nLabel=Strip\t579\tX=42241.74\ty=3658.03 \nLabel=Strip\t580\tX=42590.87\ty=3750.66 \nLabel=Strip\t581\tX=42240.29\ty=3822.77 \nLabel=Strip\t582\tX=42589.39\ty=3915.54 \nLabel=Strip\t583\tX=42238.79\ty=3987.51 \nLabel=Strip\t584\tX=42587.85\ty=4080.41 \nLabel=Strip\t585\tX=42237.21\ty=4152.24 \nLabel=Strip\t586\tX=42586.24\ty=4245.29 \nLabel=Strip\t587\tX=42235.58\ty=4316.98 \nLabel=Strip\t588\tX=42584.57\ty=4410.16 \nLabel=Strip\t589\tX=42233.88\ty=4481.72 \nLabel=Strip\t590\tX=42582.83\ty=4575.04 \nLabel=Strip\t591\tX=42232.11\ty=4646.47 \nLabel=Strip\t592\tX=42581.03\ty=4739.92 \nLabel=Strip\t593\tX=42230.29\ty=4811.21 \nLabel=Strip\t594\tX=42579.17\ty=4904.79 \nLabel=Strip\t595\tX=42228.40\ty=4975.95 \nLabel=Strip\t596\tX=42577.24\ty=5069.67 \nLabel=Strip\t597\tX=42226.44\ty=5140.69 \nLabel=Strip\t598\tX=42575.25\ty=5234.55 \nLabel=Strip\t599\tX=42224.43\ty=5305.44 \nLabel=Strip\t600\tX=42573.20\ty=5399.43 \nLabel=Strip\t601\tX=42222.34\ty=5470.18 \nLabel=Strip\t602\tX=42571.08\ty=5564.31 \nLabel=Strip\t603\tX=42220.20\ty=5634.93 \nLabel=Strip\t604\tX=42568.90\ty=5729.19 \nLabel=Strip\t605\tX=42217.99\ty=5799.67 \nLabel=Strip\t606\tX=42566.65\ty=5894.07 \nLabel=Strip\t607\tX=42215.72\ty=5964.42 \nLabel=Strip\t608\tX=42564.34\ty=6058.95 \nLabel=Strip\t609\tX=42213.38\ty=6129.16 \nLabel=Strip\t610\tX=42561.97\ty=6223.83 \nLabel=Strip\t611\tX=42210.98\ty=6293.91 \nLabel=Strip\t612\tX=42559.54\ty=6388.71 \nLabel=Strip\t613\tX=42208.52\ty=6458.66 \nLabel=Strip\t614\tX=42557.03\ty=6553.59 \nLabel=Strip\t615\tX=42205.99\ty=6623.40 \nLabel=Strip\t616\tX=42554.47\ty=6718.48 \nLabel=Strip\t617\tX=42203.40\ty=6788.15 \nLabel=Strip\t618\tX=42551.84\ty=6883.36 \nLabel=Strip\t619\tX=42200.74\ty=6952.90 \nLabel=Strip\t620\tX=42549.15\ty=7048.24 \nLabel=Strip\t621\tX=42198.02\ty=7117.65 \nLabel=Strip\t622\tX=42546.40\ty=7213.12 \nLabel=Strip\t623\tX=42195.24\ty=7282.40 \nLabel=Strip\t624\tX=42543.58\ty=7378.01 \nLabel=Strip\t625\tX=42192.40\ty=7447.14 \nLabel=Strip\t626\tX=42540.69\ty=7542.89 \nLabel=Strip\t627\tX=42189.49\ty=7611.89 \nLabel=Strip\t628\tX=42537.75\ty=7707.78 \nLabel=Strip\t629\tX=42186.51\ty=7776.64 \nLabel=Strip\t630\tX=42534.74\ty=7872.66 \nLabel=Strip\t631\tX=42183.48\ty=7941.39 \nLabel=Strip\t632\tX=42531.66\ty=8037.54 \nLabel=Strip\t633\tX=42180.38\ty=8106.14 \nLabel=Strip\t634\tX=42528.53\ty=8202.43 \nLabel=Strip\t635\tX=42177.21\ty=8270.89 \nLabel=Strip\t636\tX=42525.32\ty=8367.31 \nLabel=Strip\t637\tX=42173.99\ty=8435.64 \nLabel=Strip\t638\tX=42522.06\ty=8532.20 \nLabel=Strip\t639\tX=42170.69\ty=8600.39 \nLabel=Strip\t640\tX=42518.73\ty=8697.08 \nLabel=Strip\t641\tX=42167.34\ty=8765.14 \nLabel=Strip\t642\tX=42515.34\ty=8861.97 \nLabel=Strip\t643\tX=42163.92\ty=8929.89 \nLabel=Strip\t644\tX=42511.88\ty=9026.85 \nLabel=Strip\t645\tX=42160.44\ty=9094.63 \nLabel=Strip\t646\tX=42508.36\ty=9191.73 \nLabel=Strip\t647\tX=42156.89\ty=9259.38 \nLabel=Strip\t648\tX=42504.78\ty=9356.62 \nLabel=Strip\t649\tX=42153.28\ty=9424.13 \nLabel=Strip\t650\tX=42501.13\ty=9521.50 \nLabel=Strip\t651\tX=42149.61\ty=9588.88 \nLabel=Strip\t652\tX=42497.42\ty=9686.39 \nLabel=Strip\t653\tX=42145.87\ty=9753.63 \nLabel=Strip\t654\tX=42493.64\ty=9851.27 \nLabel=Strip\t655\tX=42142.07\ty=9918.38 \nLabel=Strip\t656\tX=42489.80\ty=10016.15 \nLabel=Strip\t657\tX=42138.20\ty=10083.13 \nLabel=Strip\t658\tX=42485.90\ty=10181.04 \nLabel=Strip\t659\tX=42134.27\ty=10247.88 \nLabel=Strip\t660\tX=42481.94\ty=10345.92 \nLabel=Strip\t661\tX=42130.28\ty=10412.62 \nLabel=Strip\t
